vi "Average_IBP_curves.vi"(0 "I in":dbl[](array[numeric]), 1 "Averaged P(B) In":dbl[][](array[numeric]), 2 "Counter":i8, 5 "Averaged I(B) In":dbl[][](array[numeric]), 7 "t in":dbl[](array[numeric]), 9 "B in":dbl[](array[numeric]), 11 "Averaged dt in":dbl[][](array[numeric]), 12 "Up/Down":bool, 13 "Sample area(mm^2)":dbl, 14 "B array":dbl[](array[numeric])) -> (4 "Averaged I(B) out":dbl[][](array[numeric]), 6 "Averaged dt Out":dbl[][](array[numeric]), 8 "Averaged P(B) Out":dbl[][](array[numeric]))   [LabVIEW 2015]
uses:
  <vilib>/Analysis/baseanly.llb/Mean (DBL).vi
  <vilib>/Analysis/NI_AALBase.lvlib
  <vilib>/gmath/NI_Gmath.lvlib
panel:
  out "yi":dbl[](array[numeric]) format="%_6g"
  out "Down":cluster{"B array":dbl[], dbl[]}(graph)
  out "XY Graph 2":cluster{"B in":dbl[], "I in":dbl[]}(graph)
  out "Up":cluster{"B array":dbl[], dbl[]}(graph)
  out "subarray 2":dbl[](array[numeric])
  out "subarray":dbl[](array[numeric])
  out "Sorted array":dbl[][](array[numeric]) format="%.5f"
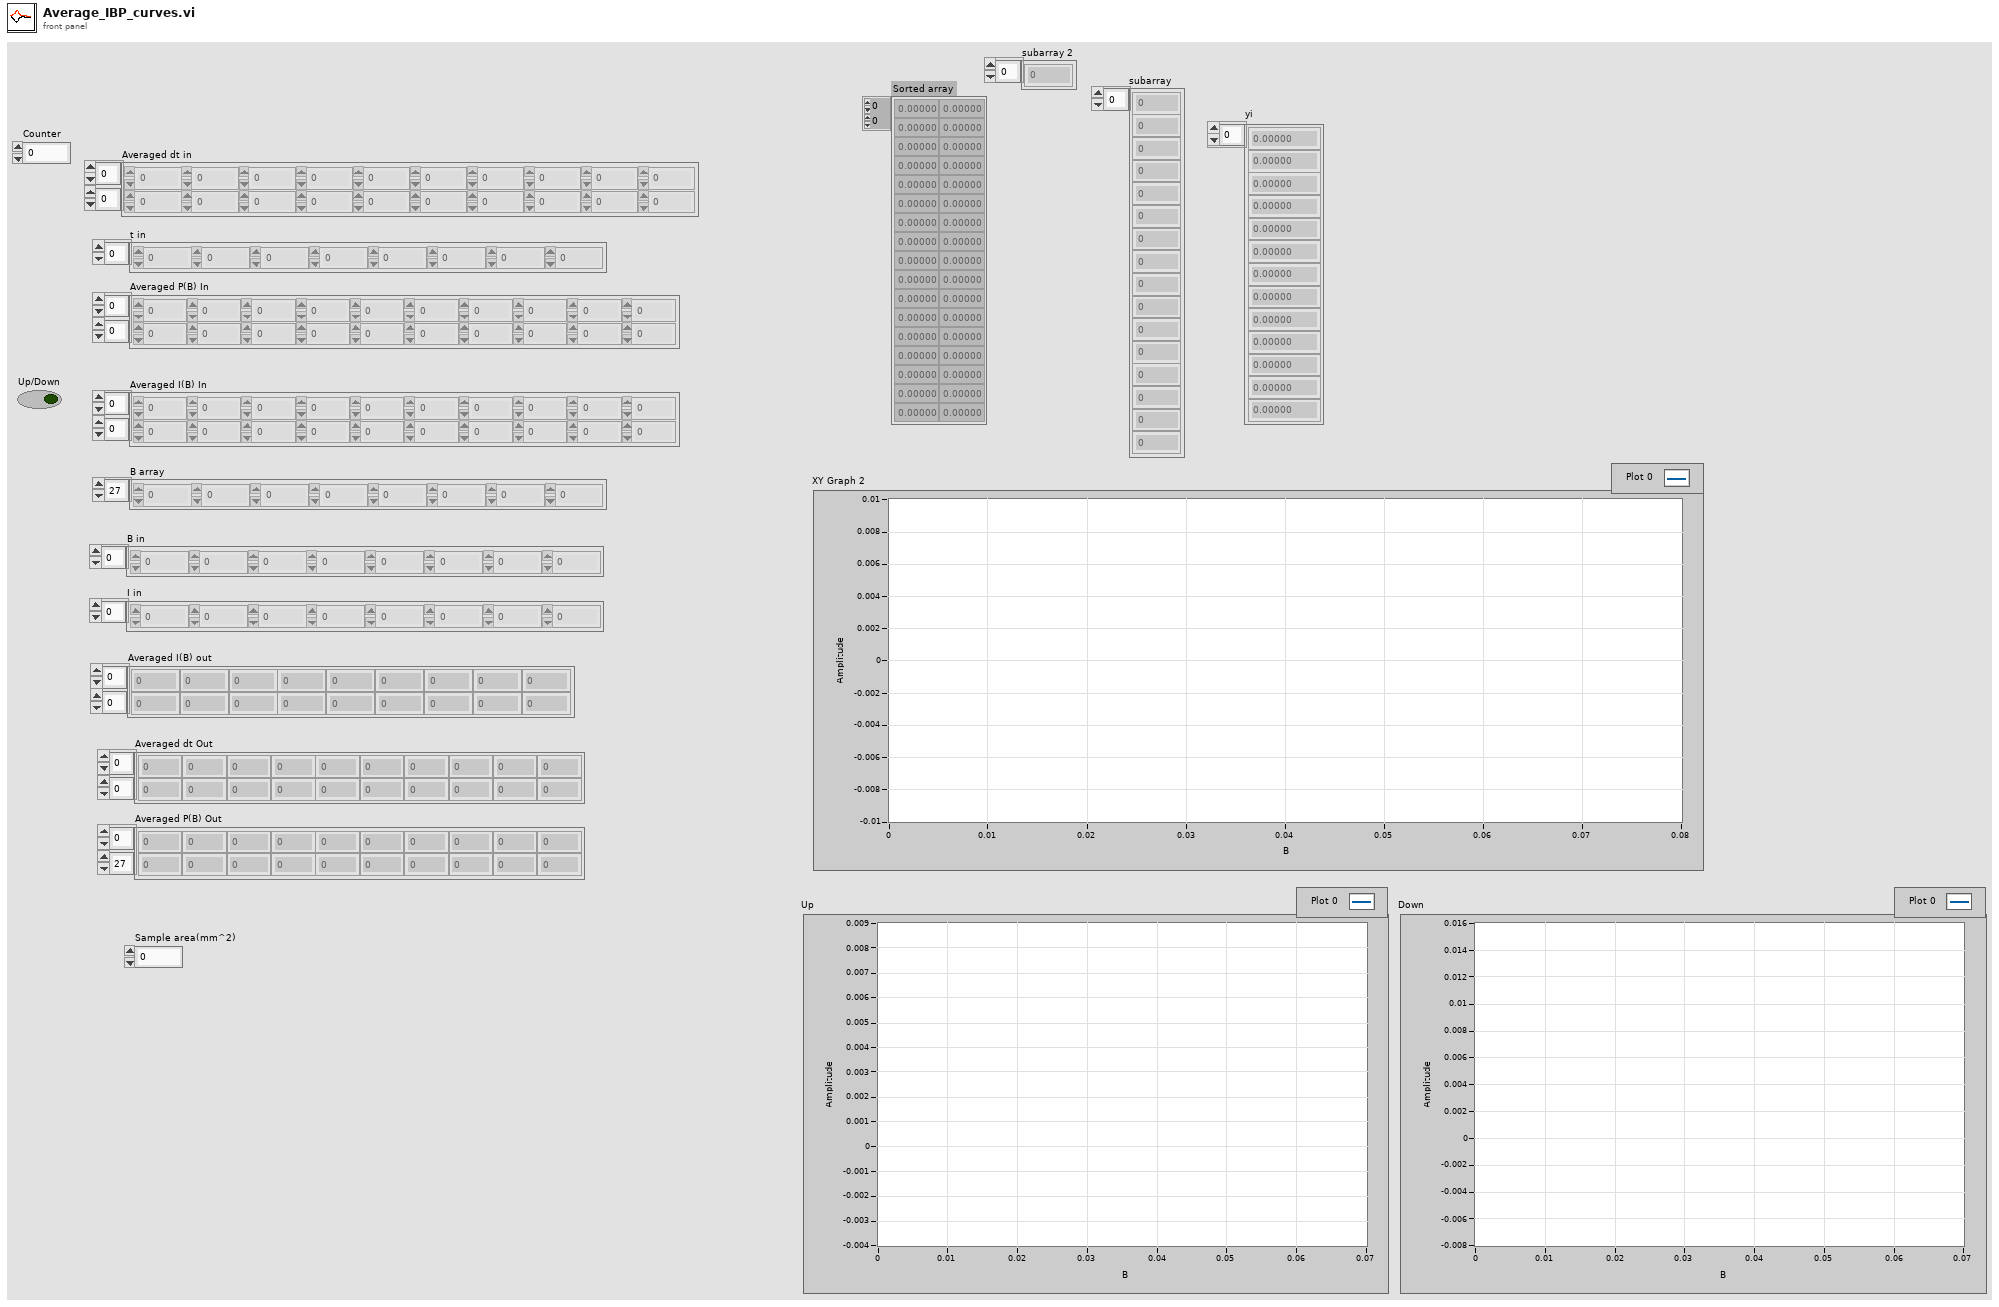
[diagram p1: front panel]
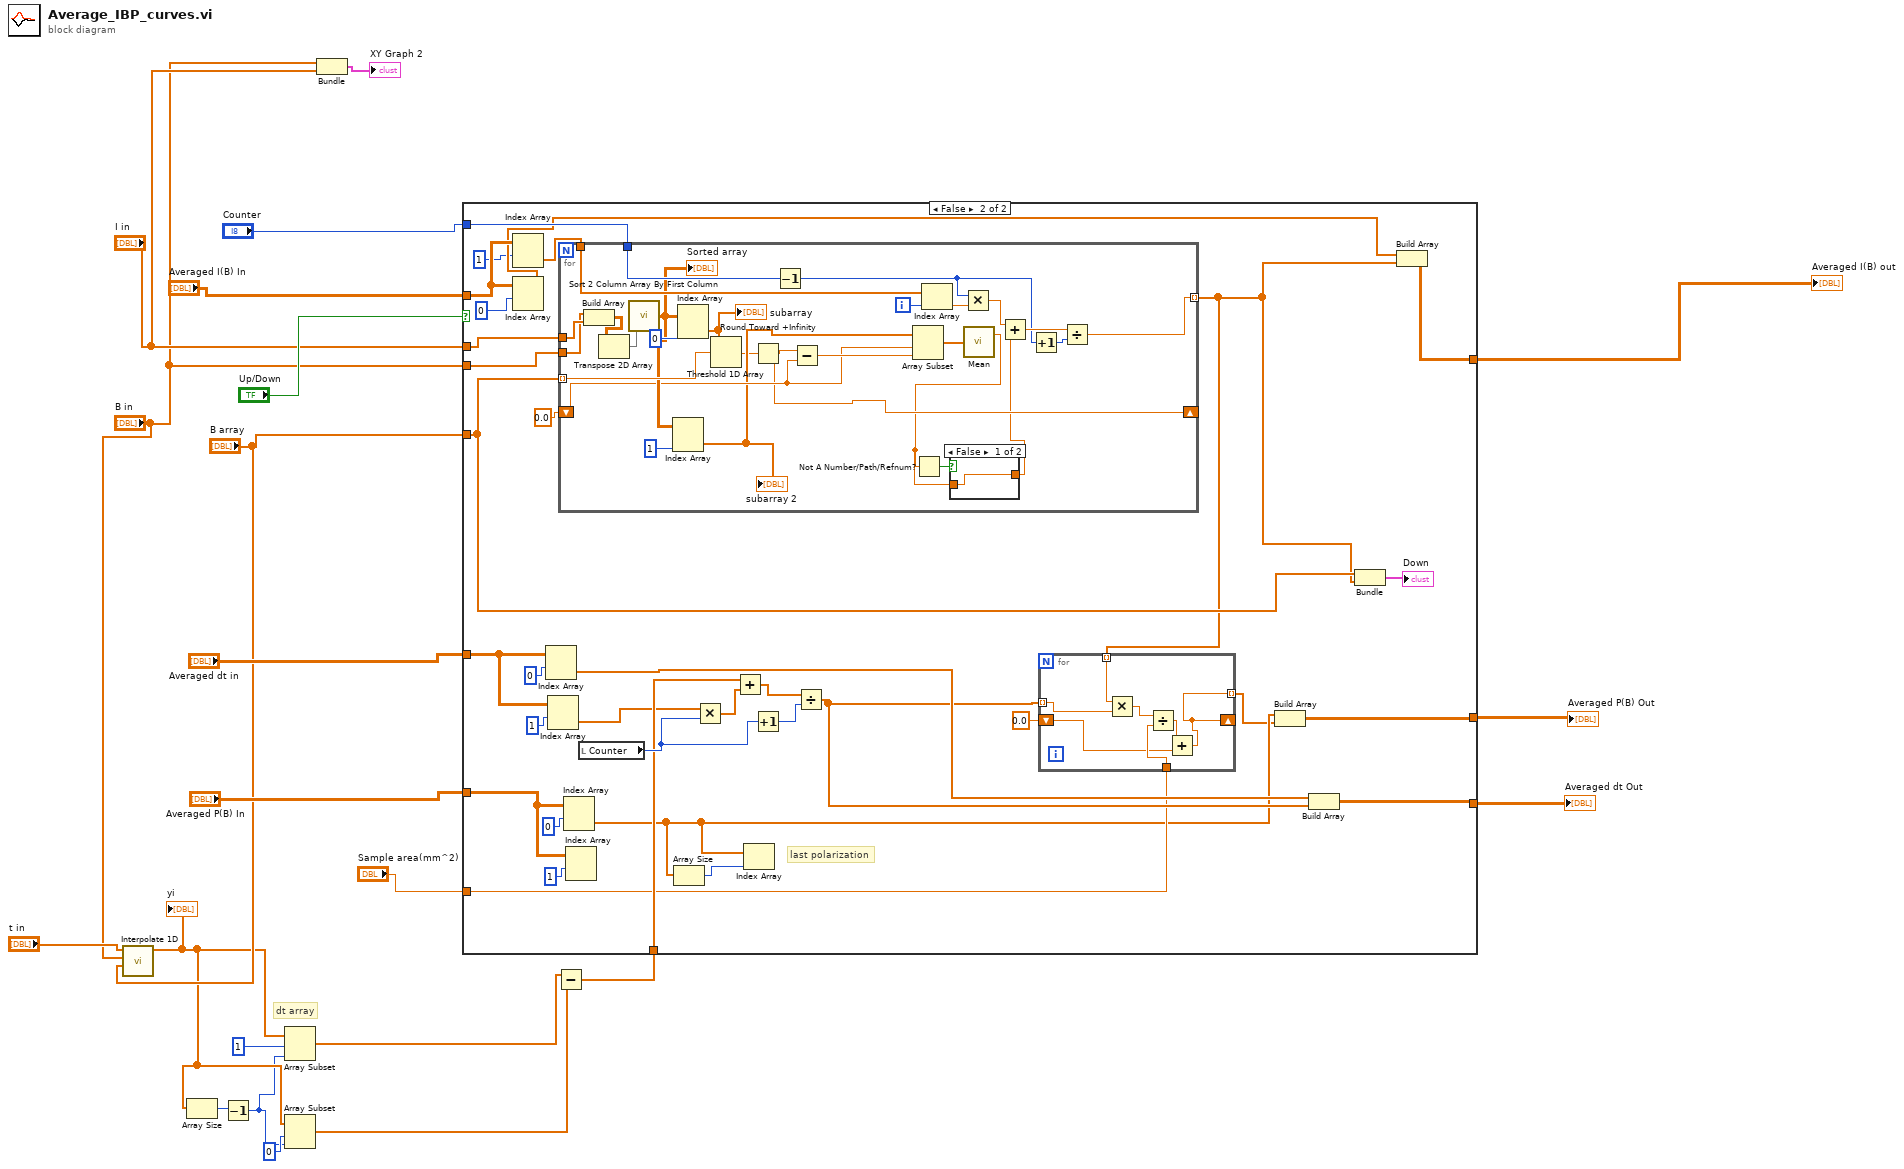
[diagram p0: block diagram]
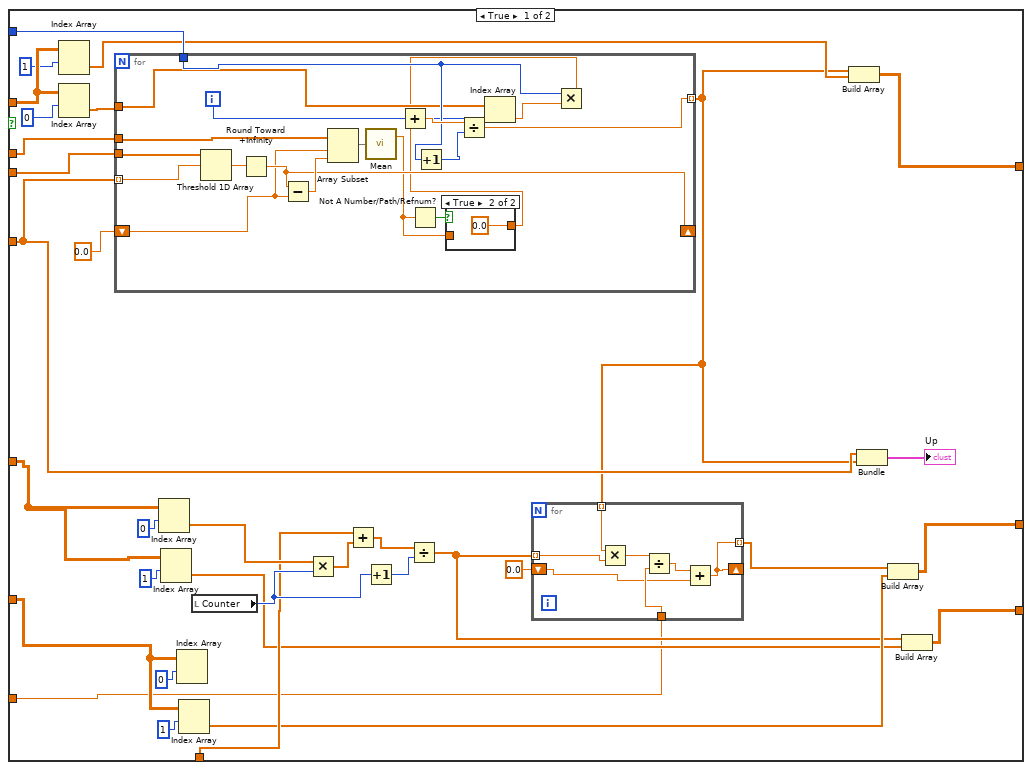
[diagram p2: hidden frame]
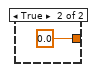
[diagram p4: hidden frame]
diagram:
  # "dt array"
  n1 = call <vilib>:"Interpolate 1D.vi"("xi"="B array", "X"="B in", "Y"="t in") -> ("yi"=w5:dbl[])  [unwired: 6 in, 2 out]
  "yi" <- w5
  n2 = Array Size(array=w5) -> (size(s)=w8:i32)
  n3 = Decrement(x=w8) -> (x-1=w1:i32)
  n4 = Array Subset(array=w5, index=1, length=w1) -> (w4:dbl[])
  n5 = Array Subset(array=w5, index=0, length=w1) -> (w3:dbl[])
  n6 = Bundle("B in"="B in", "I in"="I in") -> (→"XY Graph 2":cluster{"B in":dbl[], "I in":dbl[]})  [unwired: 1 in]
  n7 = Subtract(x=w4, y=w3) -> (x-y=w12:dbl[])
  n8 = case shown="False" "Up/Down" {
    tunnel: "Averaged I(B) In" -> [w51 w114]
    tunnel: "I in" -> [w53 w116]
    tunnel: "B in" -> [w33 w95]
    tunnel: "Counter" -> [w52 w115]
    tunnel: "B array" -> [w32 w96]
    tunnel: [w50 w113] -> w22
    tunnel: "Averaged dt in" -> [w40 w103]
    tunnel: "Averaged P(B) In" -> [w39 w102]
    tunnel: w12 -> [w38 w101]
    tunnel: [w36 w100] -> w17
    tunnel: [w34 w97] -> w16
    tunnel: "Sample area(mm^2)" -> [w23 w88]
    frame True {
      n9 = Index Array(array=w51, index (row)=1 ("disabled index (col)")) -> (element=w47:dbl[])  [unwired: 1 in]
      n10 = Index Array(array=w51, index (row)=0 ("disabled index (col)")) -> (element=w55:dbl[])  [unwired: 1 in]
      n11 = for {
        tunnel: w55 -> [w74]
        tunnel: w32 -> [w64] mode=indexing
        tunnel: w33 -> [w81]
        shift-right: [w69] -> _
        shift-left: 0.0 -> [w68]
        tunnel: w53 -> [w80]
        tunnel: w52 -> [w76]
        tunnel: [w75] -> w27 mode=indexing
        i -> [w73]
        n12 = Threshold 1D Array(2:w64, 3:w81) -> (0:w70:dbl)  [unwired: 1 in]
        n13 = Round Toward +Infinity(x=w70) -> (ceil(x): smallest int >= x=w69:dbl)
        n14 = Subtract(x=w69, y=w68) -> (x-y=w79:dbl)
        n15 = Array Subset(array=w80, index=w68, length=w79) -> (w71:dbl[])
        n16 = call-poly <vilib>:"Mean.vi"("X"=w71) -> ("mean"=w66:dbl)  [unwired: 1 out]
        n17 = Not A Number/Path/Refnum?(number/path/refnum=w66) -> (NaN/Path/Refnum?=w67:bool)
        n18 = Increment(x=w76) -> (x+1=w77:i8)
        n19 = case shown="True" w67 {
          tunnel: [w82 0.0] -> w65
          tunnel: w66 -> [w82 _]
          frame False {
          }
          frame True {
          }
        }
        n20 = Index Array(array=w74, index=w73) -> (element=w72:dbl)
        n21 = Multiply(x=w76, y=w72) -> (x*y=w63:dbl)
        n22 = Add(x=w63, y=w65) -> (x+y=w78:dbl)
        n23 = Divide(x=w78, y=w77) -> (x/y=w75:dbl)
      }
      n24 = Index Array(array=w40, index (row)=0 ("disabled index (col)")) -> (element=w41:dbl[])  [unwired: 1 in]
      n25 = Index Array(array=w40, index (row)=1 ("disabled index (col)")) -> (element=w35:dbl[])  [unwired: 1 in]
      n26 = Index Array(array=w39, index (row)=0 ("disabled index (col)")) -> ()  [unwired: 1 in, 1 out]
      n27 = Index Array(array=w39, index (row)=1 ("disabled index (col)")) -> (element=w37:dbl[])  [unwired: 1 in]
      n28 = local read "Counter"() -> (w43:i8)
      n29 = Multiply(x=w41, y=w43) -> (x*y=w42:dbl[])
      n30 = Add(x=w38, y=w42) -> (x+y=w44:dbl[])
      n31 = Increment(x=w43) -> (x+1=w45:i8)
      n32 = Divide(x=w44, y=w45) -> (x/y=w26:dbl[])
      n33 = for {
        shift-right: [w57] -> _
        shift-left: 0.0 -> [w56]
        tunnel: [w57] -> w24 mode=indexing
        tunnel: w27 -> [w62] mode=indexing
        tunnel: w26 -> [w61] mode=indexing
        tunnel: w23 -> [w60]
        n34 = Multiply(x=w62, y=w61) -> (x*y=w59:dbl)
        n35 = Divide(x=w59, y=w60) -> (x/y=w58:dbl)
        n36 = Add(x=w58, y=w56) -> (x+y=w57:dbl)
      }
      n37 = Build Array(w27, w47) -> (w50:dbl[][])
      n38 = Bundle("B array"=w32, w27) -> (→"Up":cluster{"B array":dbl[], dbl[]})  [unwired: 1 in]
      n39 = Build Array(w24, w37) -> (w36:dbl[][])
      n40 = Build Array(w26, w35) -> (w34:dbl[][])
    }
    frame False {
      # "last polarization"
      n41 = Index Array(array=w114, index (row)=1 ("disabled index (col)")) -> (element=w112:dbl[])  [unwired: 1 in]
      n42 = Index Array(array=w114, index (row)=0 ("disabled index (col)")) -> (element=w111:dbl[])  [unwired: 1 in]
      n43 = Index Array(array=w103, index (row)=0 ("disabled index (col)")) -> (element=w98:dbl[])  [unwired: 1 in]
      n44 = Index Array(array=w103, index (row)=1 ("disabled index (col)")) -> (element=w99:dbl[])  [unwired: 1 in]
      n45 = for {
        tunnel: w112 -> [w145]
        tunnel: w96 -> [w151] mode=indexing
        tunnel: w95 -> [w140]
        shift-right: [w130] -> _
        shift-left: 0.0 -> [w133]
        tunnel: w116 -> [w141]
        tunnel: w115 -> [w146]
        tunnel: [w125] -> w89 mode=indexing
        i -> [w144]
        n46 = Build Array(w140, w141) -> (w135:dbl[][])
        n47 = Transpose 2D Array(2D array=w135) -> (transposed array=w134:dbl[][])
        n48 = call "Sort 2 Column Array By First Column.vi"("2D array to sort"=w134) -> ("Sorted array"=w137:dbl[][])
        "Sorted array" <- w137
        n49 = Index Array(array=w137, index (col)=1 ("disabled index (col)")) -> (element=w132:dbl[])  [unwired: 1 in]
        "subarray 2" <- w132
        n50 = Index Array(array=w137, index (col)=0 ("disabled index (col)")) -> (element=w139:dbl[])  [unwired: 1 in]
        "subarray" <- w139
        n51 = Threshold 1D Array(2:w151, 3:w139) -> (0:w131:dbl)  [unwired: 1 in]
        n52 = Round Toward +Infinity(x=w131) -> (ceil(x): smallest int >= x=w130:dbl)
        n53 = Decrement(x=w146) -> (x-1=w126:i8)
        n54 = Subtract(x=w130, y=w133) -> (x-y=w150:dbl)
        n55 = Array Subset(array=w132, index=w133, length=w150) -> (w142:dbl[])
        n56 = Index Array(array=w145, index=w144) -> (element=w143:dbl)
        n57 = Multiply(x=w126, y=w143) -> (x*y=w149:dbl)
        n58 = call-poly <vilib>:"Mean.vi"("X"=w142) -> ("mean"=w128:dbl)  [unwired: 1 out]
        n59 = Not A Number/Path/Refnum?(number/path/refnum=w128) -> (NaN/Path/Refnum?=w129:bool)
        n60 = case shown="False" w129 {
          tunnel: [w152 0.0] -> w127
          tunnel: w128 -> [w152 _]
          frame False {
          }
          frame True {
          }
        }
        n61 = Add(x=w149, y=w127) -> (x+y=w148:dbl)
        n62 = Increment(x=w126) -> (x+1=w147:i8)
        n63 = Divide(x=w148, y=w147) -> (x/y=w125:dbl)
      }
      n64 = Index Array(array=w102, index (row)=0 ("disabled index (col)")) -> (element=w87:dbl[])  [unwired: 1 in]
      n65 = Index Array(array=w102, index (row)=1 ("disabled index (col)")) -> ()  [unwired: 1 in, 1 out]
      n66 = local read "Counter"() -> (w105:i8)
      n67 = Array Size(array=w87) -> (size(s)=w86:i32)
      n68 = Multiply(x=w99, y=w105) -> (x*y=w104:dbl[])
      n69 = Add(x=w101, y=w104) -> (x+y=w106:dbl[])
      n70 = Index Array(array=w87, index=w86) -> ()  [unwired: 1 out]
      n71 = Increment(x=w105) -> (x+1=w107:i8)
      n72 = Divide(x=w106, y=w107) -> (x/y=w90:dbl[])
      n73 = for {
        tunnel: w90 -> [w123] mode=indexing
        tunnel: w89 -> [w122] mode=indexing
        shift-right: [w120] -> _
        shift-left: 0.0 -> [w118]
        tunnel: [w120] -> w84 mode=indexing
        tunnel: w88 -> [w119]
        n74 = Multiply(x=w122, y=w123) -> (x*y=w124:dbl)
        n75 = Divide(x=w124, y=w119) -> (x/y=w121:dbl)
        n76 = Add(x=w121, y=w118) -> (x+y=w120:dbl)
      }
      n77 = Build Array(w87, w84) -> (w100:dbl[][])
      n78 = Build Array(w98, w90) -> (w97:dbl[][])
      n79 = Bundle("B array"=w96, w89) -> (→"Down":cluster{"B array":dbl[], dbl[]})  [unwired: 1 in]
      n80 = Build Array(w111, w89) -> (w113:dbl[][])
    }
  }
  "Averaged I(B) out" <- w22
  "Averaged P(B) Out" <- w17
  "Averaged dt Out" <- w16
